vi "ActivationFunction.vi"(2 "x":dbl) -> (0 "y":dbl)   [LabVIEW 2013]
doc: "Computes activation function (sigmoid)"
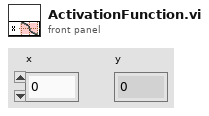
[diagram p1: front panel]
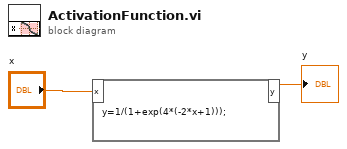
[diagram p0: block diagram]
diagram:
  n1 = formula code="y=1/(1+exp(4*(-2*x+1)));"("x"="x") -> ("y"=→"y":dbl)
